vi "BooleanOperators.vi"() -> ()   [LabVIEW 2018]
panel:
  out "XOR":bool
  out "OR":bool
  out "AND":bool
  in  "Input 2":bool
  in  "Input 1":bool
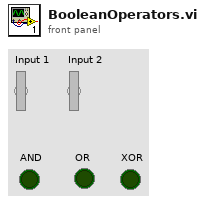
[diagram p1: front panel]
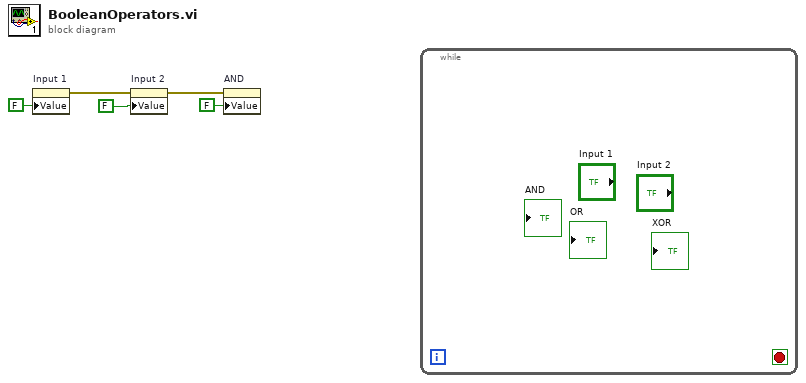
[diagram p0: block diagram]
diagram:
  n1 = property on="Input 1" class="Bool (strict)"("Value"=FALSE ("Input 1")) -> (error out=w3:errorcluster)  [unwired: 2 in, 1 out]
  n2 = property on="Input 2" class="Bool (strict)"(error in=w3, "Value"=FALSE ("Input 2")) -> (error out=w2:errorcluster)  [unwired: 1 in, 1 out]
  n3 = property on="AND" class="Bool (strict)"(error in=w2, "Value"=FALSE ("AND")) -> ()  [unwired: 1 in, 2 out]
  n4 = while {
    stop <- _ stop-if-true
  }
